vi "Purge Dialog.vi"(8 "error in":errorcluster, 11 "Potting Procedure in":refnum<class "Potting Procedure.lvclass">) -> (0 "error out":errorcluster, 2 "Canceled":bool, 3 "Potting Procedure out":refnum<class "Potting Procedure.lvclass">)   [LabVIEW 2011]
uses:
  Procedure Classes/Potting Procedure/Potting Procedure.lvclass
  Shared Components/Config Manager Class/Type Definitions/Named Position.ctl
  Shared Components/Gantry Class/Gantry Class.lvclass
  Procedure Classes/Potting Procedure/Type Definitions/Purge.ctl
panel:
  in  "activate dispenser":bool
  in  "OK Button":bool
  in  "Cancel Button":bool
  # "Now you need to Purge the Needle. \nHere are instructions!\n    Step 1: Purge it!\n    Step 2: ???\n    Step 3: Profit!\n\nClick \"OK\" when you are finished."
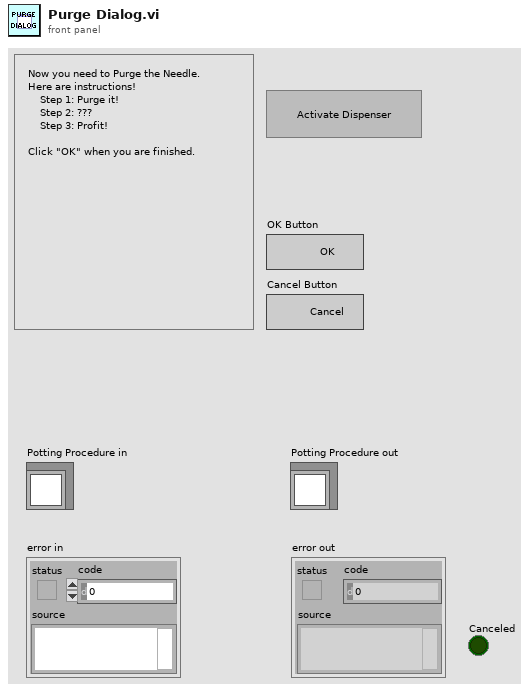
[diagram p1: front panel]
types:
  T1 = enum8{"Enabled", "Disabled", "Disabled and Grayed Out"}
  T2 = typedef "Named Position.ctl" = enum16{"home", "module_chuck_0", "module_chuck_1", "module_chuck_2", "module_chuck_3", "module_chuck_4", "glue_reservoir_chuck", "stamp_tool_chuck", "weight_tool_chuck", "needle_calibration", "tool_rack_pos_0_in", "tool_rack_pos_0_out", "tool_rack_pos_1_in", "tool_rack_pos_1_out", "tool_rack_pos_2_in", "tool_rack_pos_2_out", "front_load_position"}
  T3 = typedef "Purge.ctl" = cluster{"Has Been Run?":bool}
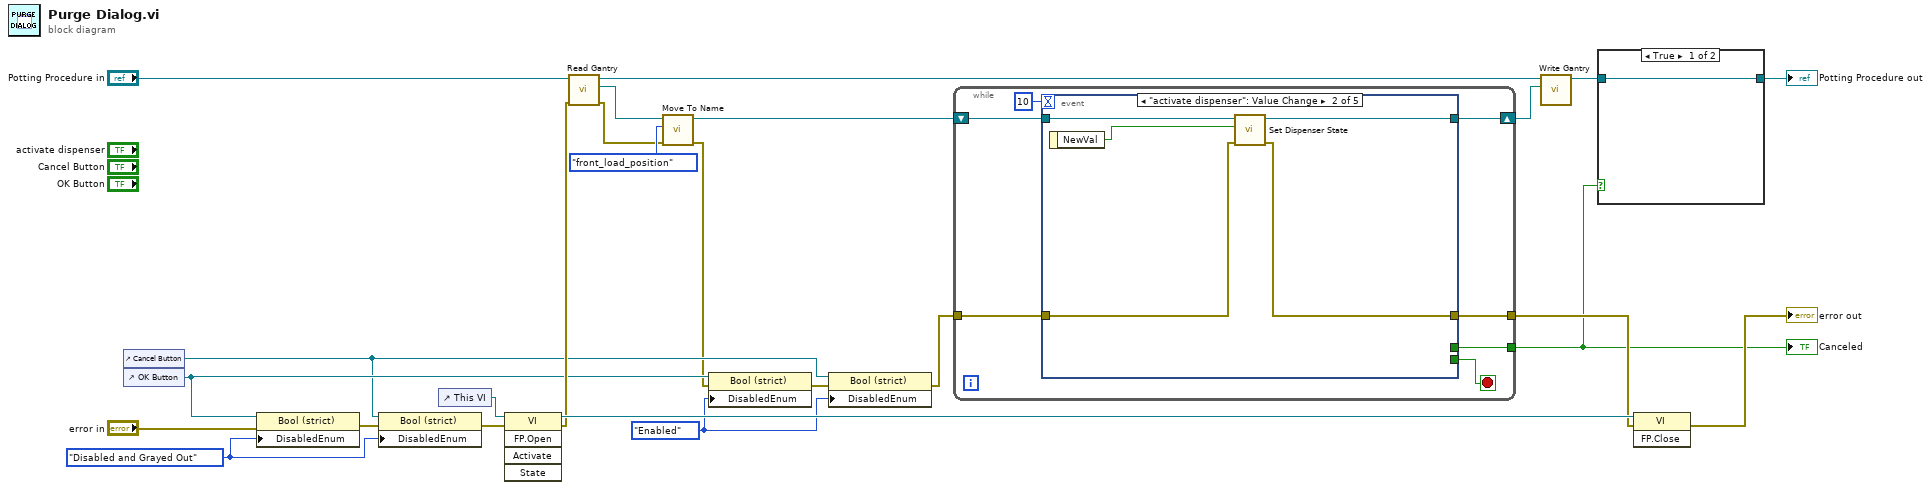
[diagram p0: block diagram]
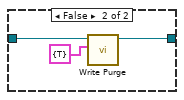
[diagram p2: hidden frame]
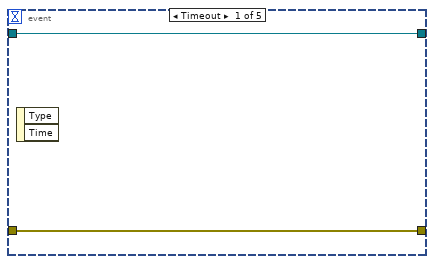
[diagram p3: hidden frame]
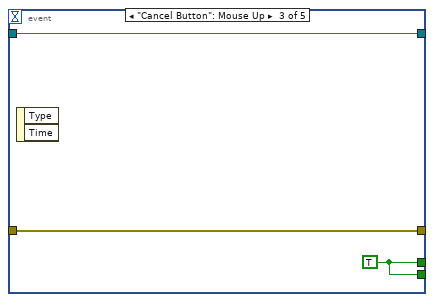
[diagram p4: hidden frame]
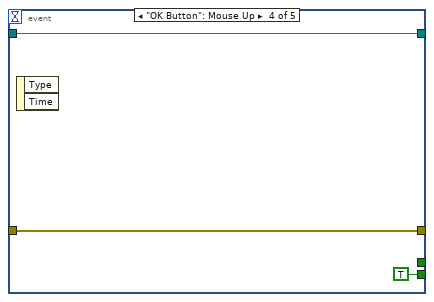
[diagram p5: hidden frame]
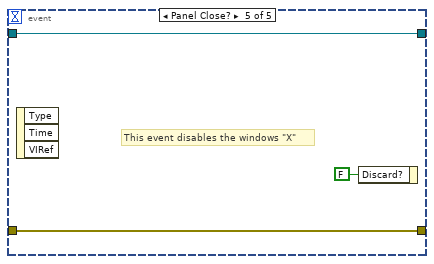
[diagram p6: hidden frame]
diagram:
  w11 = T1."Enabled" ("Disabled")
  w16 = T1."Disabled and Grayed Out" ("Disabled")
  n1 = control-ref of="Cancel Button"() -> (w9:refnum<vi>)
  n2 = control-ref of="OK Button"() -> (w10:refnum<vi>)
  n3 = property class="Bool (strict)"(reference=w10, error in="error in", "DisabledEnum"=w16) -> (error out=w18:errorcluster)  [unwired: 1 out]
  n4 = property class="Bool (strict)"(reference=w9, error in=w18, "DisabledEnum"=w16) -> (error out=w15:errorcluster)  [unwired: 1 out]
  n5 = control-ref of="This VI"() -> (w25:refnum<vi>)
  n6 = invoke class="VI" method="FP.Open"(reference=w25, error in=w15) -> (reference out=w24:refnum<vi>, error out=w14:errorcluster)  [unwired: 3 in, 3 out]
  n7 = call-dynamic "Read Gantry.vi"("error in (no error)"=w14, "Potting Procedure in"="Potting Procedure in") -> ("error out"=w13:errorcluster, "Gantry"=w19:refnum<class "Gantry Class.lvclass">, "Potting Procedure out"=w1:refnum<class "Potting Procedure.lvclass">)  [unwired: 7 in]
  n8 = call-dynamic "Move To Name.vi"("error in"=w13, "Destination"=Named_Position."front_load_position", "Gantry in"=w19) -> ("error out"=w5:errorcluster, "Gantry out"=w4:refnum<class "Gantry Class.lvclass">)  [unwired: 7 in]
  n9 = property class="Bool (strict)"(reference=w10, error in=w5, "DisabledEnum"=w11) -> (error out=w12:errorcluster)  [unwired: 1 out]
  n10 = property class="Bool (strict)"(reference=w9, error in=w12, "DisabledEnum"=w11) -> (error out=w8:errorcluster)  [unwired: 1 out]
  n11 = while {
    tunnel: [w28] -> w7
    tunnel: w8 -> [w29]
    tunnel: [w30] -> w22
    shift-right: [w26] -> w3
    shift-left: w4 -> [w27]
    stop <- w31 stop-if-true
    n12 = event shown="[1] \"activate dispenser\": Value Change" {
      selector: _ -> [_ _ _ _ _]
      dyn-events: _ -> [_ _ _ _ _]
      timeout: 10 -> [_ _ _ _ _]
      tunnel: [_ _ w41 TRUE _] -> w31
      tunnel: [w34 w35 w42 w45 w47] -> w30
      tunnel: w29 -> [w34 w36 w42 w45 w47]
      tunnel: [_ _ w41 _ _] -> w28
      tunnel: w27 -> [w33 w39 w40 w43 w46]
      tunnel: [w33 w38 w40 w43 w46] -> w26
      event Timeout {
        n13 = event-data() -> ()  [unwired: 1 in, 2 out]
      }
      event "activate dispenser": Value Change {
        n14 = event-data() -> ("NewVal"=w37:bool)  [unwired: 1 in]
        n15 = call-dynamic "Set Dispenser State.vi"("error in"=w36, "On/Off"=w37, "Gantry in"=w39) -> ("error out"=w35:errorcluster, "Gantry out"=w38:refnum<class "Gantry Class.lvclass">)  [unwired: 7 in]
      }
      event "Cancel Button": Mouse Up {
        w41 = TRUE
        n16 = event-data() -> ()  [unwired: 1 in, 2 out]
      }
      event "OK Button": Mouse Up {
        n17 = event-data() -> ()  [unwired: 1 in, 2 out]
      }
      event Panel Close? {
        # "This event disables the windows \"X\""
        n18 = event-data() -> ()  [unwired: 1 in, 3 out]
        n19 = event-data("Discard?"=FALSE) -> ()  [unwired: 1 in, 1 out]
      }
    }
  }
  "Canceled" <- w7
  n20 = call-dynamic "Write Gantry.vi"("Gantry"=w3, "Potting Procedure in"=w1) -> ("Potting Procedure out"=w2:refnum<class "Potting Procedure.lvclass">)  [unwired: 8 in, 1 out]
  n21 = case shown="True" w7 {
    tunnel: w2 -> [w49 w52]
    tunnel: [w49 w51] -> w6
    frame True {
    }
    frame False {
      n22 = call-dynamic "Write Purge.vi"("Purge"=T3 {"Has Been Run?"=TRUE}, "Potting Procedure in"=w52) -> ("Potting Procedure out"=w51:refnum<class "Potting Procedure.lvclass">)  [unwired: 8 in, 1 out]
    }
  }
  "Potting Procedure out" <- w6
  n23 = invoke class="VI" method="FP.Close"(reference=w24, error in=w22) -> (error out=→"error out":errorcluster)  [unwired: 1 in, 2 out]
